vi "getWallError.vi"(11 "segments":T1(array[cluster])) -> (2 "verticalErros":dbl[](array[numeric]), 3 "horizontalErrors":dbl[](array[numeric]))   [LabVIEW 2015]
panel:
  out "verticalCorse":cluster{"X":sgl, "Y":sgl}[](array[cluster])=[{"X"=-400.0, "Y"=600.0}, {"X"=-200.0, "Y"=600.0}, {"X"=0.0, "Y"=600.0}, {"X"=200.0, "Y"=600.0}, {"X"=400.0, "Y"=600.0}]
  out "hoizontalCorse":cluster{"X":sgl, "Y":sgl}[](array[cluster])=[{"X"=-400.0, "Y"=600.0}, {"X"=-200.0, "Y"=600.0}, {"X"=0.0, "Y"=600.0}, {"X"=200.0, "Y"=600.0}, {"X"=400.0, "Y"=600.0}]
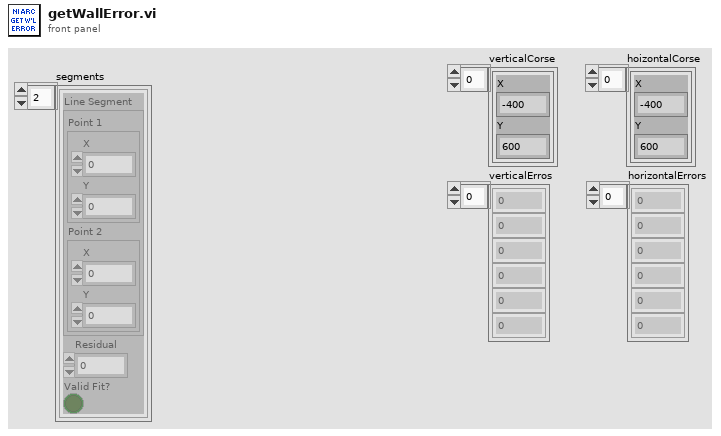
[diagram p1: front panel]
types:
  T1 = cluster{"Line Segment":cluster{"Point 1":cluster{"X":sgl, "Y":sgl}, "Point 2":cluster{"X":sgl, "Y":sgl}}, "Residual":dbl, "Valid Fit?":bool}[]
  T2 = cluster{"Point 1":cluster{"X":sgl, "Y":sgl}, "Point 2":cluster{"X":sgl, "Y":sgl}}
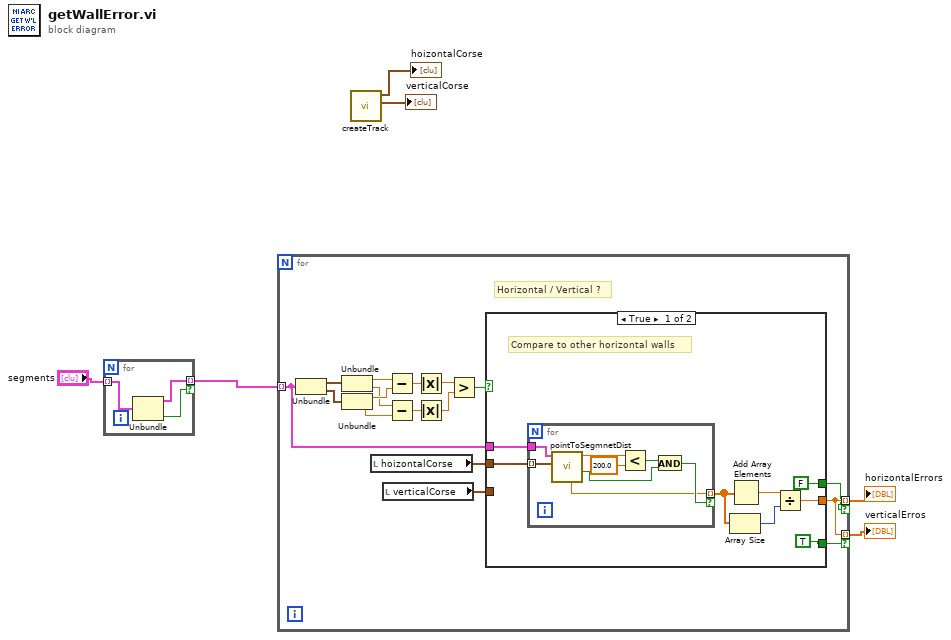
[diagram p0: block diagram]
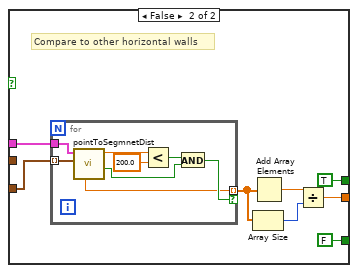
[diagram p2: hidden frame]
diagram:
  n1 = for {
    tunnel: "segments" -> [w9] mode=indexing
    tunnel: [w7] -> w4 mode=indexing if=w8
    n2 = Unbundle(w9) -> ("Line Segment"=w7:T2, "Valid Fit?"=w8:bool)  [unwired: 1 out]
  }
  n3 = for {
    tunnel: w4 -> [w14] mode=indexing
    tunnel: [w12] -> w5 mode=indexing if=w10
    tunnel: [w12] -> w3 mode=indexing if=w11
    # "Horizontal / Vertical ?"
    n4 = Unbundle(w14) -> ("Point 1"=w26:cluster{"X":sgl, "Y":sgl}, "Point 2"=w25:cluster{"X":sgl, "Y":sgl})
    n5 = Unbundle(w26) -> ("X"=w24:sgl, "Y"=w22:sgl)
    n6 = Unbundle(w25) -> ("X"=w23:sgl, "Y"=w21:sgl)
    n7 = local read "hoizontalCorse"() -> (w15:cluster{"X":sgl, "Y":sgl}[])
    n8 = local read "verticalCorse"() -> (w13:cluster{"X":sgl, "Y":sgl}[])
    n9 = Subtract(x=w24, y=w23) -> (x-y=w20:sgl)
    n10 = Subtract(x=w22, y=w21) -> (x-y=w19:sgl)
    n11 = Absolute Value(x=w20) -> (abs(x)=w17:sgl)
    n12 = Absolute Value(x=w19) -> (abs(x)=w18:sgl)
    n13 = Greater?(x=w17, y=w18) -> (0:w16:bool)
    n14 = case shown="True" w16 {
      tunnel: w15 -> [w34 _]
      tunnel: w14 -> [w33 w50]
      tunnel: [w29 w46] -> w12
      tunnel: w13 -> [_ w45]
      tunnel: [TRUE FALSE] -> w11
      tunnel: [FALSE TRUE] -> w10
      frame True {
        # "Compare to other horizontal walls"
        n15 = for {
          tunnel: w34 -> [w42] mode=indexing
          tunnel: w33 -> [w41]
          tunnel: [w35] -> w32 mode=indexing if=w37
          n16 = call "pointToSegmnetDist.vi"("point"=w42, "Line Segment"=w41) -> ("onSegment"=w36:bool, "distance"=w40:dbl, "y-dist"=w35:dbl)  [unwired: 5 in, 2 out]
          n17 = Less?(x=w40, y=200.0) -> (x < y?=w38:bool)
          n18 = And(x=w38, y=w36) -> (x .and. y?=w37:bool)
        }
        n19 = Array Size(array=w32) -> (size(s)=w30:i32)
        n20 = Add Array Elements(numeric array=w32) -> (sum=w31:dbl)
        n21 = Divide(x=w31, y=w30) -> (x/y=w29:dbl)
      }
      frame False {
        # "Compare to other horizontal walls"
        n22 = for {
          tunnel: w45 -> [w53] mode=indexing
          tunnel: w50 -> [w54]
          tunnel: [w55] -> w49 mode=indexing if=w56
          n23 = call "pointToSegmnetDist.vi"("point"=w53, "Line Segment"=w54) -> ("onSegment"=w51:bool, "distance"=w52:dbl, "x-Dist"=w55:dbl)  [unwired: 5 in, 2 out]
          n24 = Less?(x=w52, y=200.0) -> (x < y?=w57:bool)
          n25 = And(x=w57, y=w51) -> (x .and. y?=w56:bool)
        }
        n26 = Array Size(array=w49) -> (size(s)=w47:i32)
        n27 = Add Array Elements(numeric array=w49) -> (sum=w48:dbl)
        n28 = Divide(x=w48, y=w47) -> (x/y=w46:dbl)
      }
    }
  }
  "horizontalErrors" <- w5
  "verticalErros" <- w3
  n29 = call "createTrack.vi"() -> ("verticalCourse"=→"verticalCorse":cluster{"X":sgl, "Y":sgl}[], "hoizontalCourse"=→"hoizontalCorse":cluster{"X":sgl, "Y":sgl}[])  [unwired: 9 in, 1 out]
